vi "cw_4_7.vi"() -> ()   [LabVIEW 2022 SP3]
panel:
  out "is valid?":bool
  in  "Password":string
  # "At min: 8 chars, 1 capital letter, 1 special char"
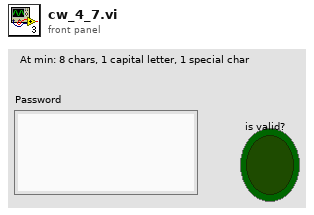
[diagram p1: front panel]
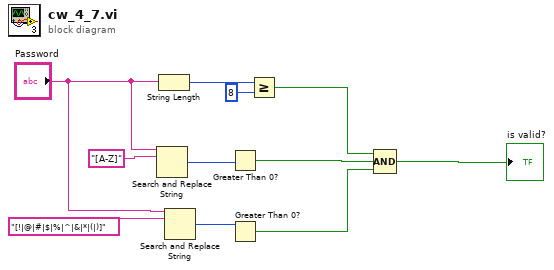
[diagram p0: block diagram]
diagram:
  n1 = Search and Replace String(input string="Password", search string="[A-Z]" ("regular expression")) -> (number of replacements=w9:i32)  [unwired: 6 in, 3 out]
  n2 = String Length(string="Password") -> (length=w11:i32)
  n3 = Search and Replace String(input string="Password", search string="[!|@|#|$|%|^|&|*|(|)]") -> (number of replacements=w7:i32)  [unwired: 6 in, 3 out]
  n4 = Greater Than 0?(x=w9) -> (x > 0?=w3:bool)
  n5 = Greater Than 0?(x=w7) -> (x > 0?=w2:bool)
  n6 = Greater Or Equal?(x=w11, y=8) -> (x >= y?=w4:bool)
  n7 = Compound Arithmetic op=AND(w4, w3, w2) -> (→"is valid?":bool)
